vi "Constant - Number of Analog Channel Numbers.vi"() -> (3 "Maximum Channel":i32=16)   [LabVIEW 2021]
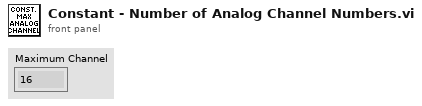
[diagram p1: front panel]
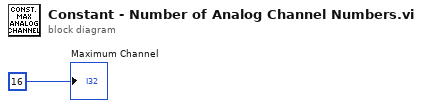
[diagram p0: block diagram]
diagram:
  "Maximum Channel" <- u16 16 ("remote port or service name")
